vi "Destroy.vi"(8 "error in (no error)":errorcluster, 11 "Skeleton in":refnum<class "Skeleton.lvclass">) -> (0 "error out":errorcluster)   [LabVIEW 2016, in "Skeleton.lvlib" / "Skeleton.lvclass"]
uses:
  Skeleton.lvclass
  Skeleton.lvclass/Skeleton.ctl
  Active Thread Configuration.ctl
  DemoSkeleton/DemoSkeleton.lvlib
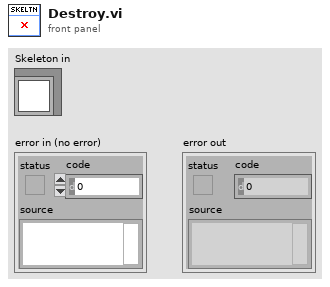
[diagram p1: front panel]
types:
  T1 = typedef "Skeleton.lvlib/Skeleton.lvclass/Private Data.ctl" = cluster{"DLL path":path, "Active Thread Map":variant}
  T2 = typedef "Skeleton.lvlib/Skeleton.lvclass/Active Thread Configuration.ctl" = cluster{"Operation":string, "Handle":u64, "LVUserEvent CallBack Reference":refnum<user-event>}
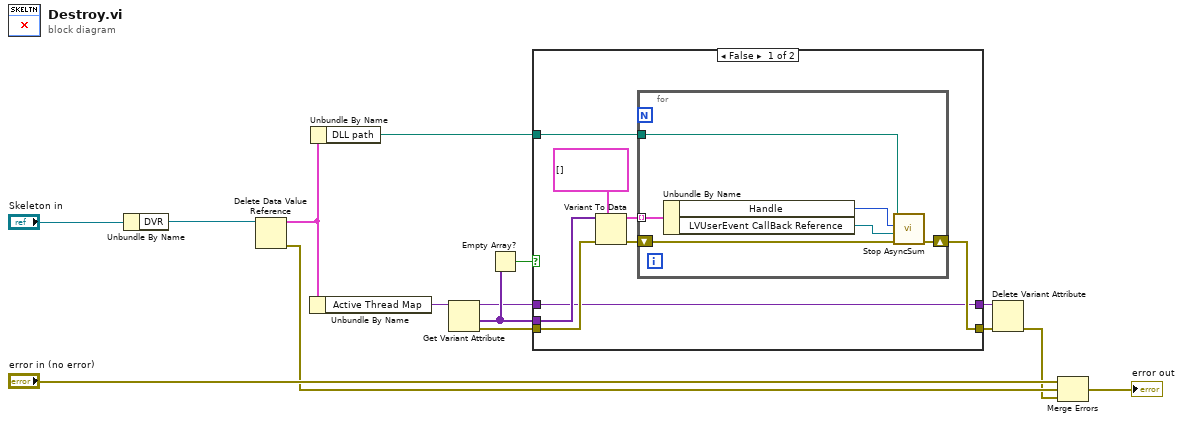
[diagram p0: block diagram]
diagram:
  n1 = Unbundle By Name("Skeleton in") -> ("DVR"=w14:refnum<data-value>)
  n2 = Delete Data Value Reference(data value reference=w14) -> (data value=w9:T1, error out=w11:errorcluster)  [unwired: 1 in]
  n3 = Unbundle By Name(w9) -> ("Active Thread Map"=w10:variant)
  n4 = Unbundle By Name(w9) -> ("DLL path"=w8:path)
  n5 = Get Variant Attribute(Variant=w10) -> (duplicate Variant=w2:variant, values=w4:variant[], error out=w7:errorcluster)  [unwired: 3 in, 1 out]
  n6 = Empty Array?(array=w4) -> (empty?=w3:bool)
  n7 = case shown="False" w3 {
    tunnel: w8 -> [w22 _]
    tunnel: w7 -> [w19 w31]
    tunnel: [w18 w31] -> w6
    tunnel: w4 -> [w17 _]
    tunnel: w2 -> [w16 w30]
    tunnel: [w16 w30] -> w1
    frame False {
      n8 = Variant To Data(error in=w19, type=T2[] [], Variant=w17) -> (data=w20:T2[], error out=w21:errorcluster)
      n9 = for {
        tunnel: w22 -> [w28]
        tunnel: w20 -> [w27] mode=indexing
        shift-right: [w24] -> w18
        shift-left: w21 -> [w29]
        n10 = Unbundle By Name(w27) -> ("Handle"=w26:u64, "LVUserEvent CallBack Reference"=w25:refnum<user-event>)
        n11 = call "Stop AsyncSum.vi"("error in (no error)"=w29, "LVUserEventCallBackRef"=w25, "Handle"=w26, "path in"=w28) -> ("error out"=w24:errorcluster)  [unwired: 6 in, 1 out]
      }
    }
    frame True {
    }
  }
  n12 = Delete Variant Attribute(4:w6, 7:w1) -> (0:w5:errorcluster)  [unwired: 1 in, 2 out]
  n13 = Merge Errors("error in (no error)", w11, w5) -> (→"error out":errorcluster)
